vi "Device-UI.vi"() -> ()   [LabVIEW 2017]
uses:
  D:/upwork/Laser Measurement Tool/Laser/tests/KIM101/Thorlabs.MotionControl.Controls.dll
  Thorlabs.MotionControl.Controls.dll
  D:/upwork/Laser Measurement Tool/Laser/tests/KIM101/Thorlabs.MotionControl.KCube.InertialMotorCLI.dll
  Thorlabs.MotionControl.KCube.InertialMotorCLI.dll
panel:
  out "CreateDevice":bool
  in  "channel":i32(ring)=1 items=["Channel1"=1, "Channel2"=2, "Channel3"=3, "Channel4"=4]
  out "GetPosition":i32
  in  "stop":bool
  in  "SerialNumber":string="97000001"
  in  "KCubeInertialMotorControl":refnum<k24>(container)
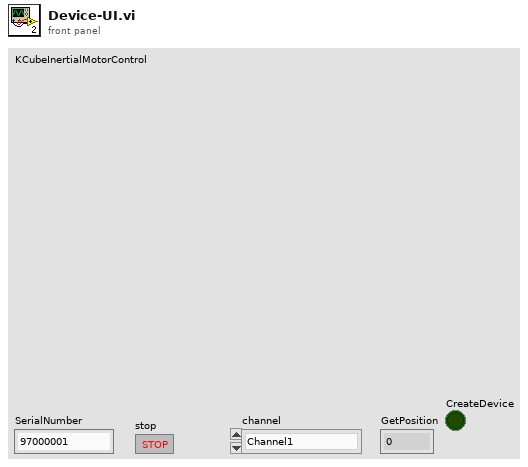
[diagram p1: front panel]
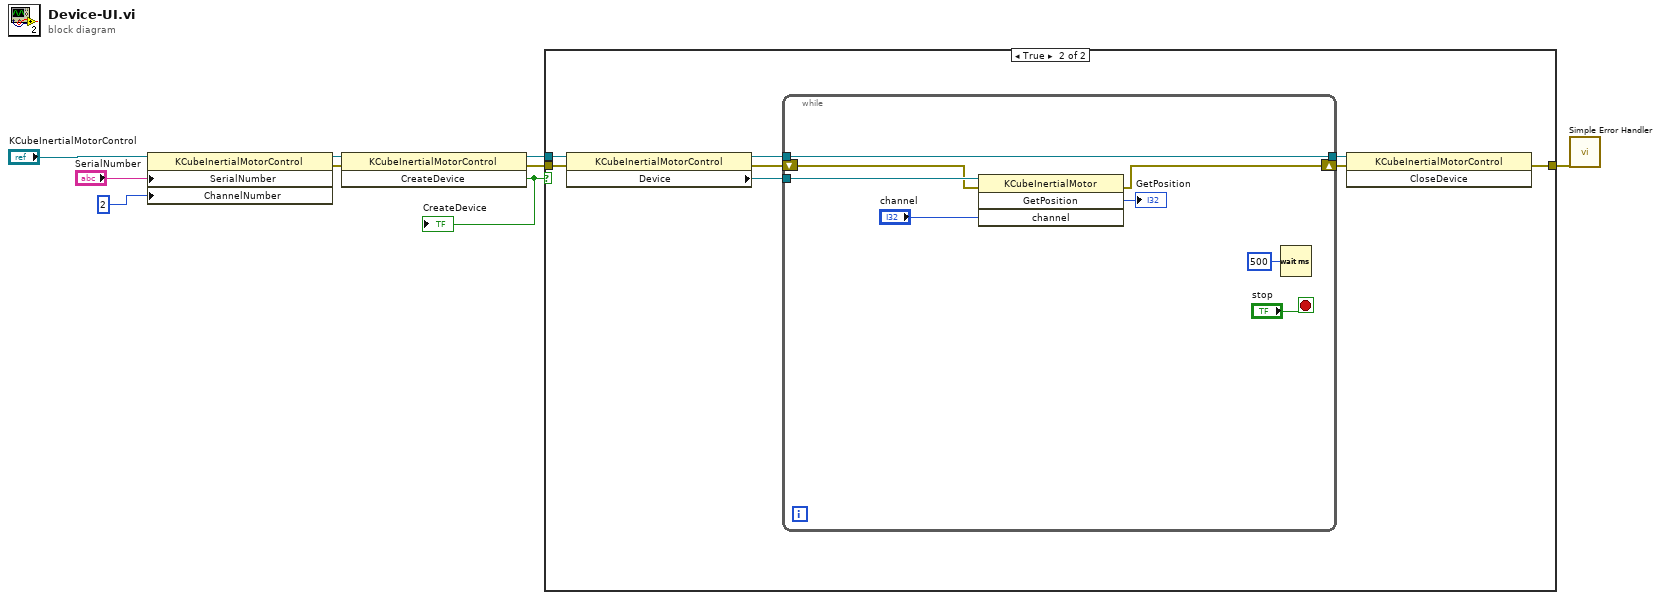
[diagram p0: block diagram]
diagram:
  n1 = property class="KCubeInertialMotorControl"(reference="KCubeInertialMotorControl", "SerialNumber"="SerialNumber", "ChannelNumber"=2) -> (reference out=w7:refnum<k24>, error out=w4:errorcluster)  [unwired: 1 in]
  n2 = invoke class="KCubeInertialMotorControl" method="CreateDevice"(reference=w7, error in=w4) -> (reference out=w6:refnum<k24>, error out=w2:errorcluster, "CreateDevice"=w3:bool)  [unwired: 1 in]
  "CreateDevice" <- w3
  n3 = case shown="True" w3 {
    tunnel: w6 -> [_ w16]
    tunnel: w2 -> [w10 w17]
    tunnel: [w10 w11] -> w1
    frame False {
    }
    frame True {
      n4 = property class="KCubeInertialMotorControl"(reference=w16, error in=w17) -> (reference out=w14:refnum<k24>, error out=w13:errorcluster, "Device"=w15:refnum<k24>)
      n5 = while {
        tunnel: w15 -> [w24]
        shift-right: [w22] -> w12
        shift-left: w13 -> [w23]
        tunnel: w14 -> [w26]
        tunnel: [w26] -> w18
        stop <- "stop" stop-if-true
        n6 = invoke class="KCubeInertialMotor" method="GetPosition"(reference=w24, error in=w23, "channel"="channel") -> (error out=w22:errorcluster, "GetPosition"=→"GetPosition":i32)  [unwired: 1 in, 2 out]
        n7 = Wait (ms)(milliseconds to wait=u32 500) -> ()  [unwired: 1 out]
      }
      n8 = invoke class="KCubeInertialMotorControl" method="CloseDevice"(reference=w18, error in=w12) -> (error out=w11:errorcluster)  [unwired: 1 in, 2 out]
    }
  }
  n9 = call <vilib>:"Simple Error Handler.vi"("error in (no error)"=w1) -> ()  [unwired: 4 in, 5 out]
